vi "tcp_udp_client-final.vi"() -> ()   [LabVIEW 2013]
doc: "The UDP protocol differs from TCP in that there is no error-checking with the packets of information that are sent, and thus no guarantee whatsoever that an intended recipient will actually receive a given piece of data.\n\nUDP does offer the ability to \"broadcast\" data across a network--simply specify an IP Address of all ones (255.255.255.255) to attempt to broadcast information network-wide. Keep in mind that routers and other network hardware will generally refuse to forward the broadcast beyond certain points, so the extent of the broadcast will in practice be limited."
uses:
  <vilib>/Utility/file.llb/Write To Spreadsheet File (DBL).vi
panel:
  out "STOP LED":bool
  in  "TCP data":bool
  out "Waveform Graph":dbl[](graph)
  out "Received Data":dbl(graph)
  in  "Stop":bool
  # "Overview: Demonstrates the use of the UDP functions to receive data over a UDP connection.\nInstructions:\n1. Ensure Simple UDP - Sender.vi is already running.\n2. Run the VI.\n3. Click Stop to stop the VI."
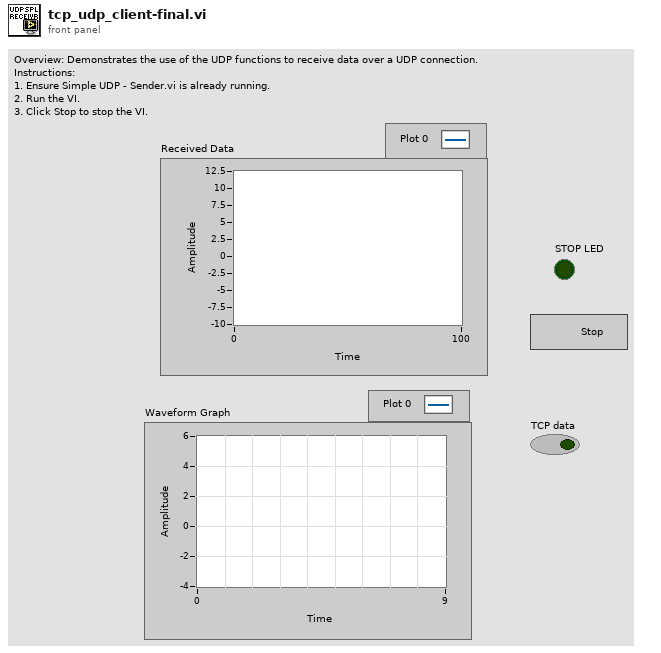
[diagram p1: front panel]
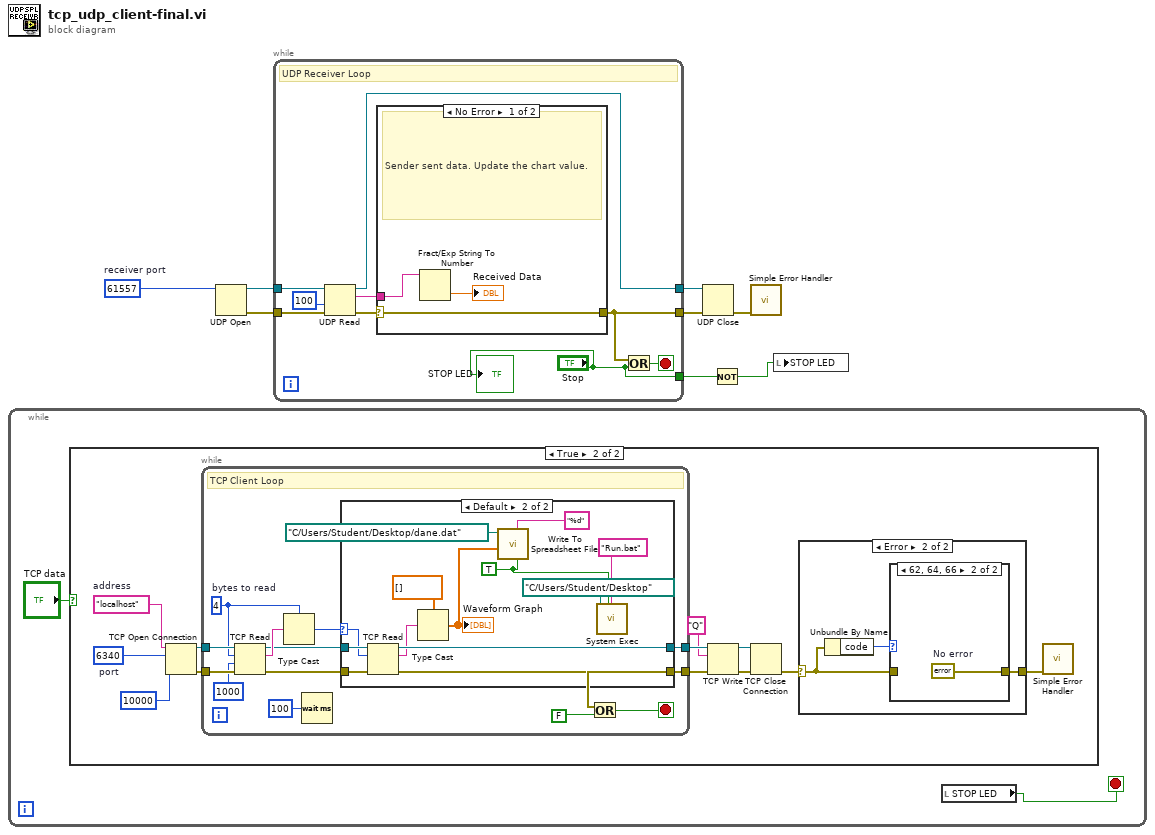
[diagram p0: block diagram]
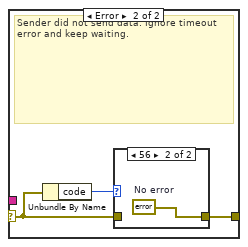
[diagram p6: hidden frame]
diagram:
  w3 = u16 61557  # receiver port
  n1 = while {
    stop <- w9 stop-if-true
    n2 = case shown="True" "TCP data" {
      frame False {
      }
      frame True {
        w12 = u16 6340  # port
        w13 = "localhost"  # address
        n3 = TCP Open Connection(address=w13, remote port or service name=w12, timeout ms (60000)=10000) -> (connection ID=w22:refnum<k5>, error out=w21:errorcluster)  [unwired: 2 in]
        n4 = while {
          tunnel: w21 -> [w37]
          tunnel: w22 -> [w38]
          tunnel: [w32] -> w19
          tunnel: [w31] -> w17
          stop <- w34 stop-if-true
          w36 = 4  # bytes to read
          # "TCP Client Loop"
          n5 = TCP Read(connection ID=w38, bytes to read=w36, error in (no error)=w37, 9:1000 ("timeout ms (25000)")) -> (connection ID out=w40:refnum<k5>, data out=w41:string, error out=w39:errorcluster)  [unwired: 1 in]
          n6 = Type Cast(type=w36, x=w41) -> (*(type *) &x=w30:i32)
          n7 = Wait (ms)(milliseconds to wait=u32 100) -> ()  [unwired: 1 out]
          n8 = case shown="Default" w30 {
            selector: w30 -> [_ w50]
            tunnel: w40 -> [w43 w56]
            tunnel: w39 -> [w42 w55]
            tunnel: [w43 w53] -> w32
            tunnel: [w42 w52] -> w31
            frame ..0 {
              # "The server has not written any data"
            }
            frame Default {
              w46 = TRUE ("transpose? (no:F)")
              n9 = TCP Read(connection ID=w56, bytes to read=w50, error in (no error)=w55) -> (connection ID out=w53:refnum<k5>, data out=w51:string, error out=w52:errorcluster)  [unwired: 2 in]
              n10 = Type Cast(type=dbl[] [] ("chart"), x=w51) -> (*(type *) &x=w49:dbl[])
              "Waveform Graph" <- w49
              n11 = call-poly <vilib>:"Write To Spreadsheet File.vi"("transpose? (no:F)"=w46, "format (%.3f)"="%d", "1D data"=w49, "file path (dialog if empty)"=path "C:/Users/Student/Desktop/dane.dat") -> ()  [unwired: 4 in, 1 out]
              n12 = call <vilib>:"System Exec.vi"("run minimized? (F)"=w46, "wait until completion? (T)"=w46, "working directory"=path "C:/Users/Student/Desktop", "command line"="Run.bat") -> ()  [unwired: 4 in, 4 out]
            }
          }
          n13 = Or(x=w31, y=FALSE ("Stop TCP klient")) -> (x .or. y?=w34:bool)
        }
        n14 = TCP Write(connection ID=w19, data in="Q", error in (no error)=w17) -> (connection ID out=w20:refnum<k5>, error out=w18:errorcluster)  [unwired: 2 out]
        n15 = TCP Close Connection(connection ID=w20, error in (no error)=w18) -> (error out=w15:errorcluster)  [unwired: 1 in, 1 out]
        n16 = case shown="Error" w15 {
          selector: w15 -> [w23 w25]
          tunnel: [w23 w24] -> w14
          frame No Error {
          }
          frame Error {
            n17 = Unbundle By Name(w25) -> ("code"=w26:i32)
            n18 = case shown="62, 64, 66" w26 {
              tunnel: w25 -> [w27 _]
              tunnel: [w27 w28] -> w24
              frame Default {
              }
              frame 62, 64, 66 {
                w28 = errorcluster {"status"=FALSE, "code"=0, "source"=""}  # No error
              }
            }
          }
        }
        n19 = call <vilib>:"Simple Error Handler.vi"("error in (no error)"=w14) -> ()  [unwired: 4 in, 5 out]
      }
    }
    n20 = local read "STOP LED"() -> (w9:bool)
  }
  n21 = UDP Open(11:w3) -> (port=w4:refnum<k16>, 0:w5:errorcluster)  [unwired: 4 in, 1 out]
  n22 = while {
    tunnel: w4 -> [w65]
    tunnel: [w58] -> w8
    tunnel: w5 -> [w63]
    tunnel: [w59] -> w6
    tunnel: ["Stop"] -> w2
    stop <- w64 stop-if-true
    # "UDP Receiver Loop"
    n23 = UDP Read(connection ID=w65, timeout ms (25000)=100, 8:w63) -> (data out=w61:string, error out=w60:errorcluster, 3:w58:refnum<k16>)  [unwired: 3 out]
    n24 = case shown="No Error" w60 {
      selector: w60 -> [w66 w70]
      tunnel: w61 -> [w68 _]
      tunnel: [w66 w69] -> w59
      frame No Error {
        # "Sender sent data. Update the chart value."
        n25 = Fract/Exp String To Number(string=w68) -> (number=→"Received Data":dbl)  [unwired: 3 in, 1 out]
      }
      frame Error {
        # "Sender did not send data. Ignore timeout error and keep waiting."
        n26 = Unbundle By Name(w70) -> ("code"=w71:i32)
        n27 = case shown="56" w71 {
          tunnel: w70 -> [w72 _]
          tunnel: [w72 w73] -> w69
          frame Default {
          }
          frame 56 {
            w73 = errorcluster {"status"=FALSE, "code"=0, "source"=""}  # No error
          }
        }
      }
    }
    n28 = Or(x=w59, y="Stop") -> (x .or. y?=w64:bool)
    "STOP LED" <- "Stop"
  }
  n29 = UDP Close(connection ID=w8, 8:w6) -> (error out=w7:errorcluster)  [unwired: 1 out]
  n30 = Not(x=w2) -> (.not. x?=w1:bool)
  n31 = call <vilib>:"Simple Error Handler.vi"("error in (no error)"=w7) -> ()  [unwired: 1 in, 8 out]
  n32 = local write "STOP LED"(w1) -> ()
